vi "Simulation Data_Global.vi"() -> ()   [LabVIEW 2013, in "Simulated Evaporative Cooler.lvclass"]
doc: "该全局VI中定义仿真蒸发冷却器所用的全部值。在仿真过程中，该全局VI的前面板可能被用于监控/调整参数。"
uses:
  Simulated Evaporative Cooler.lvclass
panel:
  in  "Outdoor Temperature":dbl=110.0 caption="室外温度"
  out "Water Level":dbl caption="水位"
  out "Water Valve State":bool caption="水阀状态"
  out "Indoor Temperature":dbl caption="室内温度"
  out "Fan A State":bool caption="风扇A状态"
  out "Fan B State":bool caption="风扇B状态"
  in  "Fan B Fault":bool caption="风扇B故障"
  in  "Fan A Fault":bool caption="风扇A故障"
  # "在仿真过程中，该前面板可能被用于监控/调整参数。"
  # "仿真输入"
  # "仿真输出"
  # "调整这些项以改变系统条件。"
  # "通过这些项可观察系统响应。"
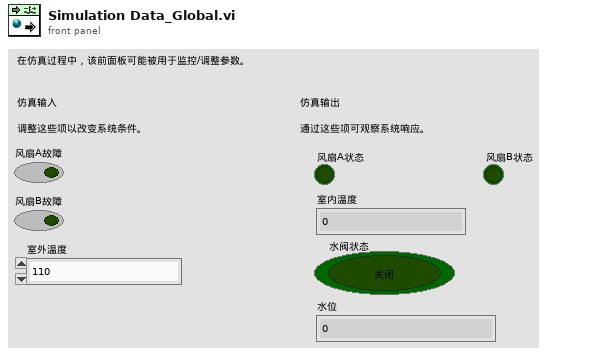
[diagram p1: front panel]
diagram:
